vi "RichToFlatni_measurementlink_sessionmanagement_v1_UnregisterMultiplexerSessionsResponse.vi"(5 "OutputClusterType":T1, 11 "InputCluster":T2) -> (3 "OutputCluster":T1)   [LabVIEW 2020, in "Measurement Plugin Session Management Client.lvlib"]
uses:
  Measurement Plugin Session Management Client.lvlib
  ni_measurementlink_sessionmanagement_v1_UnregisterMultiplexerSessionsResponse.ctl
  ni_measurementlink_sessionmanagement_v1_UnregisterMultiplexerSessionsResponse_Flat.ctl
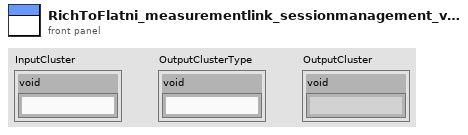
[diagram p1: front panel]
types:
  T1 = typedef "Measurement Plugin Session Management Client.lvlib/ni_measurementlink_sessionmanagement_v1_UnregisterMultiplexerSessionsResponse_Flat.ctl" = cluster{"void":string}
  T2 = typedef "Measurement Plugin Session Management Client.lvlib/ni_measurementlink_sessionmanagement_v1_UnregisterMultiplexerSessionsResponse.ctl" = cluster{"void":string}
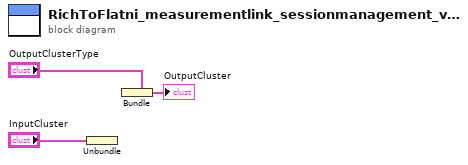
[diagram p0: block diagram]
diagram:
  n1 = Unbundle "Unbundle"("InputCluster") -> ()  [unwired: 1 out]
  n2 = Bundle "Bundle"(cluster="OutputClusterType") -> (→"OutputCluster":T1)  [unwired: 1 in]
